vi "AB_Log_Error_Usage_Data.vi"(8 "Error In":errorcluster, 10 "CEIP Key (NI_APP_BUILDER_ERROR)":T1, 11 "Build class":refnum<class>) -> (0 "Error Out":errorcluster)   [LabVIEW 2020]
uses:
  <vilib>/AppBuilder/AB_Log_Error_Usage_Data_Type.ctl
  <vilib>/UDC/Controls/LogMessageFrequency.ctl
  <vilib>/UDC/Controls/LogMessageSize.ctl
  <vilib>/UDC/niceiplib.lvlib
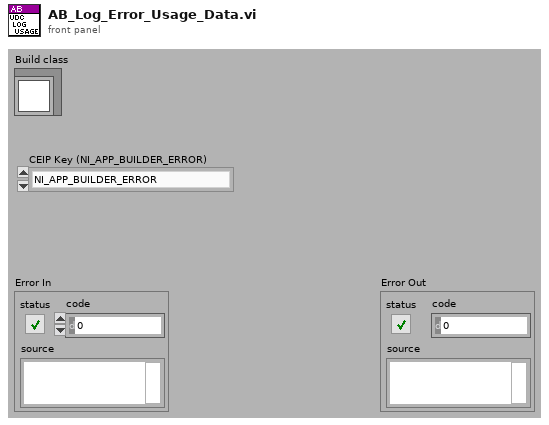
[diagram p1: front panel]
types:
  T1 = typedef "AB_Log_Error_Usage_Data_Type.ctl" = enum16{"NI_APP_BUILDER_ERROR", "NI_INSTALLER_BUILDER_ERROR"}
  T2 = typedef "niceiplib.lvlib/LogMessageFrequency.ctl" = enum32{"OncePerSession", "LowFrequency", "MediumFrequency", "HighFrequency", "KBMouseEvents"}
  T3 = typedef "niceiplib.lvlib/LogMessageSize.ctl" = enum32{"SmallMessage", "MediumMessage", "LargeMessage"}
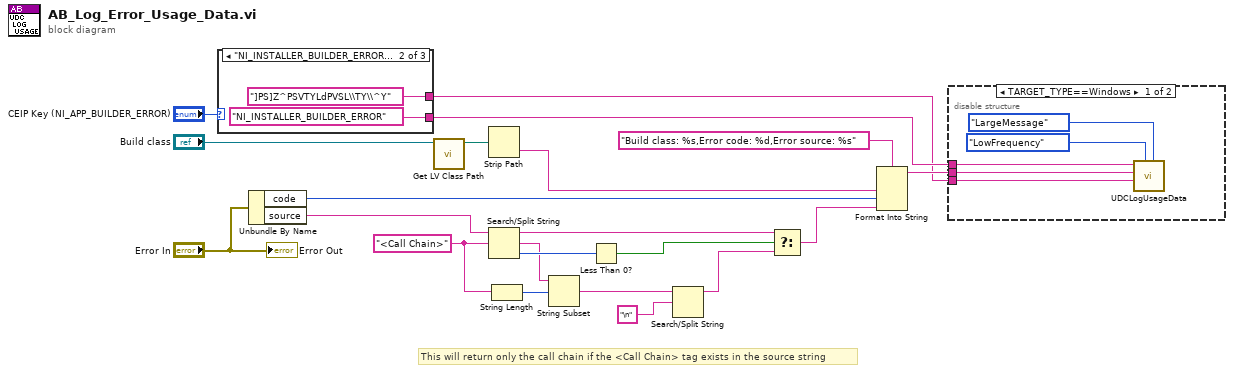
[diagram p0: block diagram]
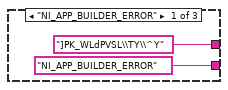
[diagram p2: hidden frame]
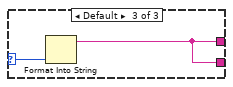
[diagram p3: hidden frame]
diagram:
  w9 = "<Call Chain>" ("string")
  # "This will return only the call chain if the <Call Chain> tag exists in the source string"
  n1 = case shown="\"NI_INSTALLER_BUILDER_ERROR\"" "CEIP Key (NI_APP_BUILDER_ERROR)" {
    selector: "CEIP Key (NI_APP_BUILDER_ERROR)" -> [_ _ w27]
    tunnel: ["]PK_WLdPVSL\\TY\\^Y" ("resulting string") "]PS]Z^PSVTYLdPVSL\\TY\\^Y" ("resulting string") w26] -> w1
    tunnel: ["NI_APP_BUILDER_ERROR" ("resulting string") "NI_INSTALLER_BUILDER_ERROR" ("resulting string") w26] -> w2
    frame "NI_APP_BUILDER_ERROR" {
    }
    frame "NI_INSTALLER_BUILDER_ERROR" {
    }
    frame Default {
      n2 = Format Into String(w27) -> (resulting string=w26:string)  [unwired: 3 in, 1 out]
    }
  }
  n3 = Unbundle By Name("Error In") -> ("code"=w17:i32, "source"=w12:string)
  n4 = call <vilib>:"Get LV Class Path.vi"("object"="Build class") -> ("class path"=w19:path)  [unwired: 9 in, 1 out]
  n5 = Strip Path(path=w19) -> (name=w18:string)  [unwired: 1 out]
  n6 = Search/Split String(string=w12, search string/char (-)=w9) -> (substring before match=w13:string, match + rest of string=w7:string, offset of match=w15:i32)  [unwired: 1 out]
  n7 = String Length(string=w9) -> (length=w8:i32)
  n8 = String Subset(string=w7, offset (0)=w8) -> (substring=w5:string)  [unwired: 1 in]
  n9 = Less Than 0?(x=w15) -> (x < 0?=w14:bool)
  n10 = Search/Split String(string=w5, search string/char (-)="\n") -> (substring before match=w4:string)  [unwired: 3 out]
  n11 = Select(t=w13, s=w14, f=w4) -> (s? t:f=w11:string)
  n12 = Format Into String(format string="Build class: %s,Error code: %d,Error source: %s", w18, w17, w11) -> (resulting string=w20:string)  [unwired: 2 in, 1 out]
  n13 = disable-structure shown="TARGET_TYPE==Windows" {
    disable-tunnel: w20 -> [w32 _]
    disable-tunnel: w2 -> [w31 _]
    disable-tunnel: w1 -> [w28 _]
    frame condition #0 (active) {
      n14 = call <vilib>:"UDCLogUsageData.vi"("LogMessageSize"=LogMessageSize."LargeMessage", "LogMessageFrequency"=LogMessageFrequency."LowFrequency", "KeyUID"=w28, "Value"=w32, "Key"=w31) -> ()  [unwired: 6 in, 1 out]
    }
    frame condition #1 {
    }
  }
  "Error Out" <- "Error In"
